vi "Test Error Handler Interface Handle Warnings.vi"(8 "error in (no error)":errorcluster, 11 "Test Case In":refnum<class "Error Handler Interface Test.lvclass">) -> (0 "error out":errorcluster, 3 "Test Case Out":refnum<class "Error Handler Interface Test.lvclass">)   [LabVIEW 2020, in "Error Handler Interface Test.lvclass"]
uses:
  Error Handler Interface Test.lvclass
  Error Handler Interface Test.lvclass/Error Handler Interface Test.ctl
  <vilib>/Astemes/LUnit/Test Case.lvclass/Test Case.ctl
  <vilib>/Astemes/LUnit/LUnit Assertion Result.lvclass/LUnit Assertion Result.ctl
  <vilib>/Astemes/LUnit/LUnit Test Case Result.lvclass/LUnit Test Case Result.ctl
  <vilib>/Astemes/LUnit/LUnit Method Result.lvclass/LUnit Method Result.ctl
  <vilib>/Astemes/LUnit/Palette/Pass If Equal.vi/cbf50e99-f124-4847-863a-8e9794d3dede.vi
  <vilib>/Astemes/LUnit/Palette/Pass.vi
  <vilib>/Astemes/LUnit/Palette/Fail.vi
  <vilib>/Astemes/LUnit/Compare Variants.vi
  <vilib>/Astemes/LUnit/Describe Comparison.vi
  <vilib>/Astemes/LUnit/Set Assertion Type.vi
  <vilib>/Astemes/LUnit/Add test result.vi
  <vilib>/Astemes/LUnit/LUnit Write Passed.vi
  <vilib>/Astemes/LUnit/LUnit Write Message.vi
  <vilib>/Astemes/LUnit/LUnit Write Description.vi
  <vilib>/Astemes/LUnit/Variant to string.vi
  <vilib>/Astemes/LUnit/LUnit Write Assertion Type.vi
  <vilib>/Astemes/LUnit/LUnit Record Assertion Result.vi
  <vilib>/Astemes/LUnit/LUnit Aggregate Assertion Results.vi
  <vilib>/Astemes/LUnit/Assertion Result/LUnit Read Status.vi
  <vilib>/Astemes/LUnit/LUnit Read Message.vi
  <vilib>/Astemes/LUnit/LUnit Read Description.vi
  <vilib>/Astemes/LUnit/Method Result/LUnit Merge Status.vi
  <vilib>/Astemes/LUnit/LUnit Concatenate result strings.vi
  <vilib>/Utility/Data Type/Get Type Information.vi
  <vilib>/Utility/LVClass/Get LV Class Name.vi
  Framework/Error Handler Interface/Error Handler Interface.lvclass
  <vilib>/Astemes/LUnit/LUnit Assertion Result.lvclass
  07e26ebd-71b7-4a78-885c-7c8051c8e292.vi
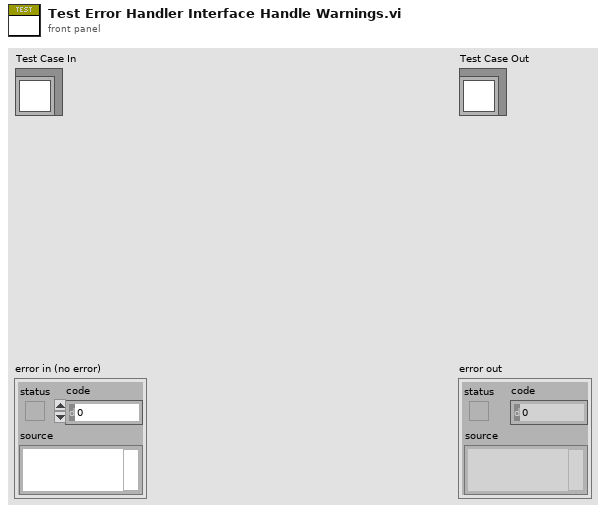
[diagram p1: front panel]
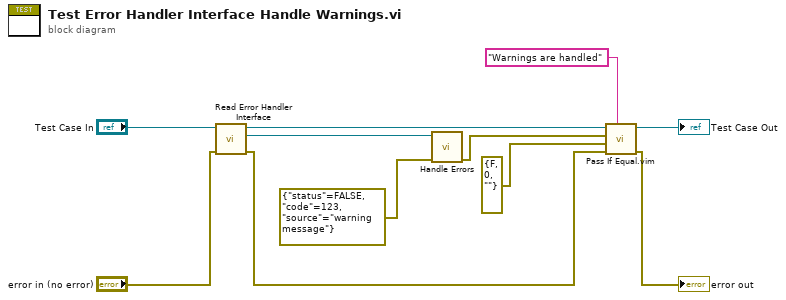
[diagram p0: block diagram]
diagram:
  n1 = call "Read Error Handler Interface.vi"("error in (no error)"="error in (no error)", "Error Handler Interface Test in"="Test Case In") -> ("error out"=w3:errorcluster, "Error Handler Interface"=w8:refnum<class "Error Handler Interface.lvclass">, "Error Handler Interface Test out"=w9:refnum<class "Error Handler Interface Test.lvclass">)  [unwired: 7 in]
  n2 = call-dynamic "Handle Errors.vi"("error in (no error)"=errorcluster {"status"=FALSE, "code"=123, "source"="warning message"}, "Error Handler Interface In"=w8) -> ("error out"=w5:errorcluster)  [unwired: 8 in, 1 out]
  n3 = call "Pass If Equal.vim"("Description"="Warnings are handled", "error in (no error)"=w3, "Actual"=errorcluster {"status"=FALSE, "code"=0, "source"=""} ("error out"), "Expected"=w5, "LUnit Test Case In"=w9) -> ("error out"=→"error out":errorcluster, "LUnit Test Case Out"=→"Test Case Out":refnum<class "Error Handler Interface Test.lvclass">)  [unwired: 5 in]
